vi "_backup hw-all.vi"() -> ()   [LabVIEW 2019]
uses:
  _ctrl/rw.ctl
  Capacitor/rc-seq_enum.ctl
  _ctrl/init-r-stop.ctl
  SubVIs/common/_ctrl/system-status.ctl
  _ctrl/Sinple-sequence-type.ctl
  SubVIs/common/hw-control.ctl
  common/UI.ctl
  _ctrl/create-rw-close.ctl
  _ctrl/start.ctl
  Devices/DL950/query type.ctl
  common/Global 1.vi
  81cc3607-908d-4f29-9377-88d8534cc897.vi
  716c5298-81ca-4b46-9759-33d23efd1b7f.vi
  5a08cc20-1eea-4034-90c3-b73213eb6239.vi
panel:
  out "appended array":dbl[](array[numeric])
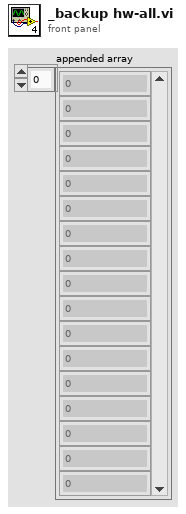
[diagram p1: front panel]
types:
  T1 = typedef "rw.ctl" = enum16{"read", "write"}
  T2 = typedef "Sinple-sequence-type.ctl" = enum16{"Register", "RC", "B1", "B2", "B3"}
  T3 = typedef "system-status.ctl" = enum16{"Initial", "Update", "Clear", "Read"}
  T4 = typedef "init-r-stop.ctl" = enum16{"ini", "read", "stop"}
  T5 = typedef "hw-control.ctl" = enum16{"DL950 ready", "DL950 clear", "DL950 trigger", "DL950 read", "DL950 read seq", "DL950 Tsingle query", "AO 12v", "AO wave", "AO 0v", "relay all-off", "Discharge check", "Discharge", "Relay1", "Relay2", "Relay3", "Relay4", "Relay5", "Relay6", "BP4610 onoff", "BP4610 set", "DSP1500 set", "DSP1500 onoff"}
  T6 = typedef "UI.ctl" = enum16{"Alarm yellow", "DL950 graph show", "DL950 graph clear", "AO value", "AO blink onoff", "Discharge relay", "Input Power", "Outpower", "Relay in1", "Relay in2", "Relay in3", "Relay in4", "Relay in5", "Relay in6", "Relay out1", "Relay out2", "Relay out3", "Relay out4", "Relay out5", "Relay out6", "Relay all off"}
  T7 = typedef "start.ctl" = enum16{"init", "open", "set", "start", "stop", "read", "read_items", "query", "close", "T_single", "reset", "exit"}
  T8 = typedef "create-rw-close.ctl" = enum16{"create", "write", "read", "close"}
  T9 = typedef "query type.ctl" = enum16{"clear", "capacitor set", "capacitor get"}
  T10 = typedef "cap_config.ctl" = cluster{"제어 전압[V]":dbl, "출력전압[V]":dbl, "전류[A]":dbl, "출력전류[A]":dbl, "ON[초]":dbl, "OFF[초]":dbl, "방전 진단[V]":dbl, "전압98[초]":dbl, "전압63[초]":dbl, "전류37[초]":dbl, "방전 시간[초]":dbl, "전압98[+/-%]":dbl, "전압63[+/-%]":dbl, "전류37[+/-%]":dbl}
  T11 = typedef "rc-seq_enum.ctl" = enum16{"hw set", "Pwr-in on", "ch-relay on", "Pwr-out on", "AO on", "AO 0v", "Pwr-in off", "Relay-all off", "Pwr-out off", "Discharge", "950 read"}
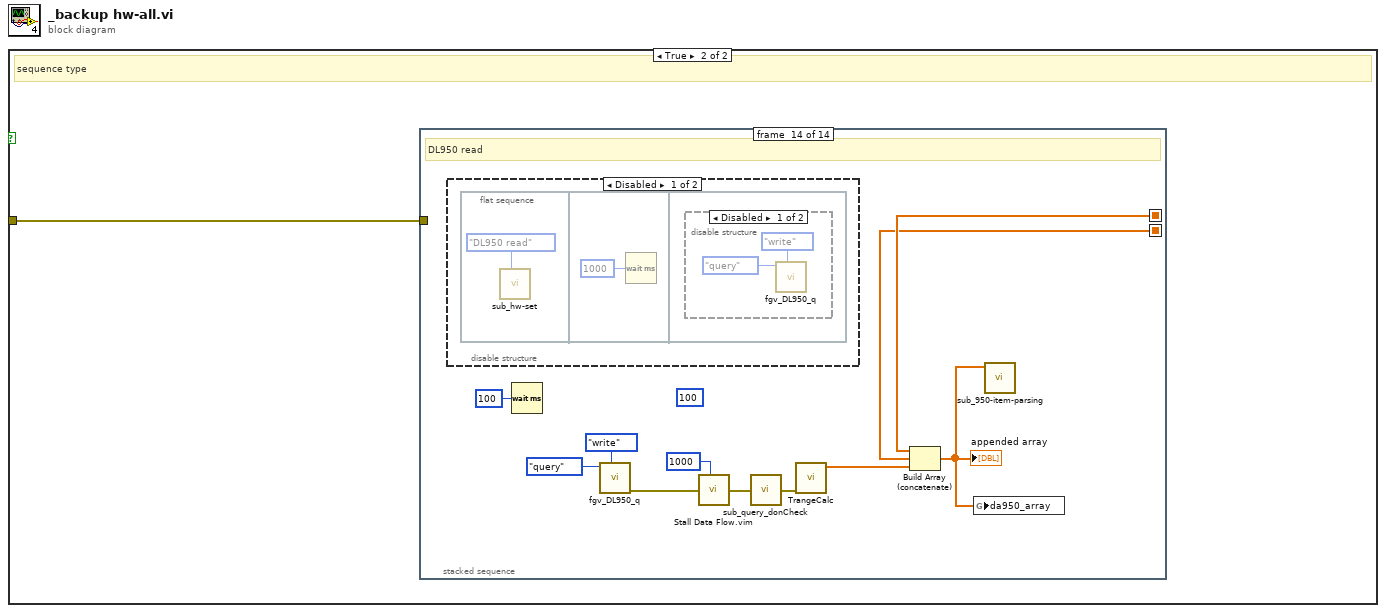
[diagram p0: block diagram]
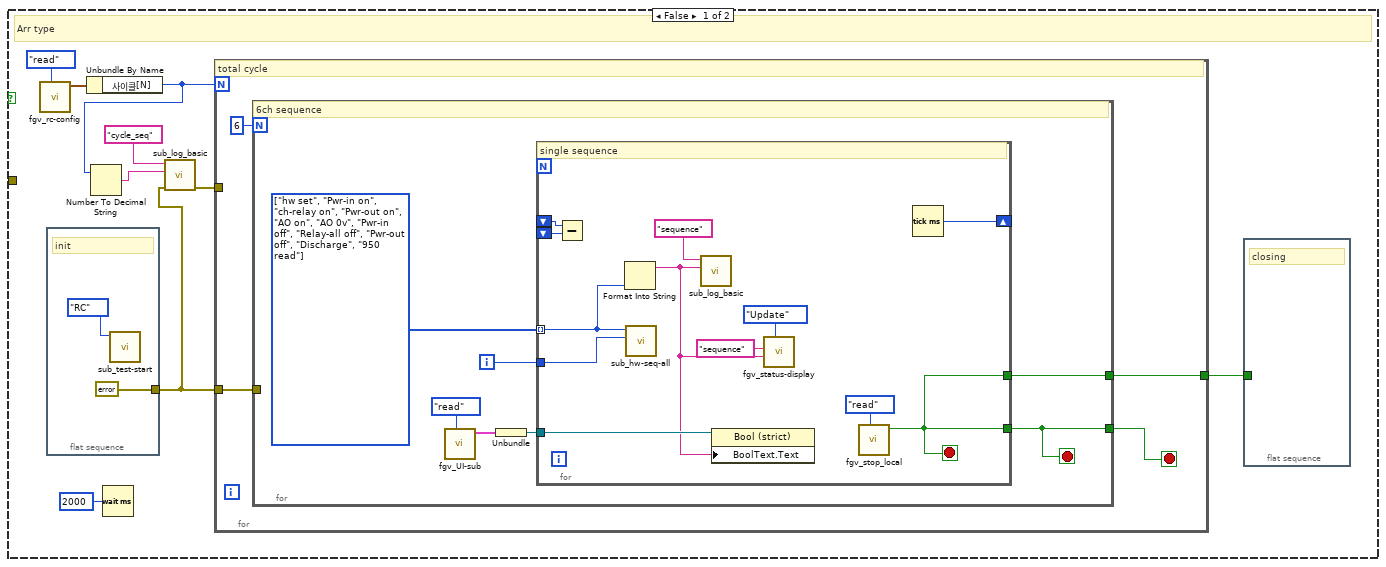
[diagram p2: hidden frame]
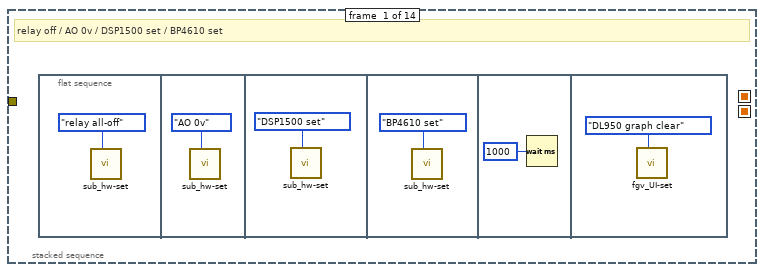
[diagram p3: hidden frame]
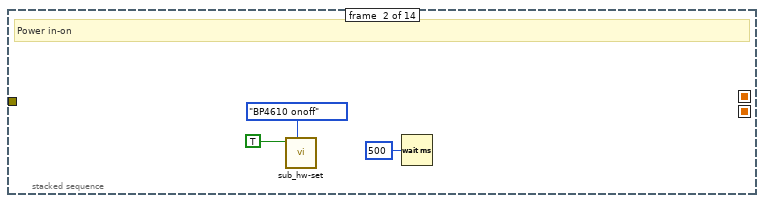
[diagram p4: hidden frame]
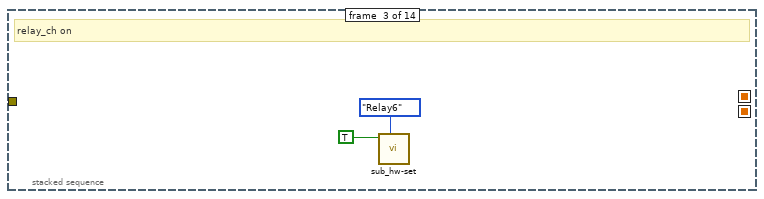
[diagram p5: hidden frame]
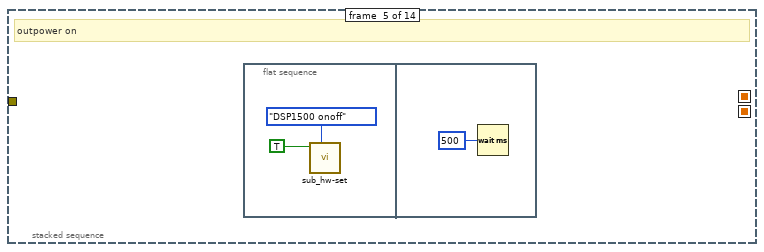
[diagram p7: hidden frame]
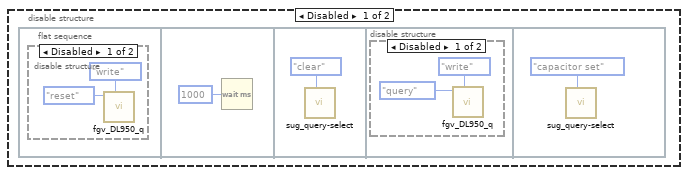
[diagram p9: hidden frame]
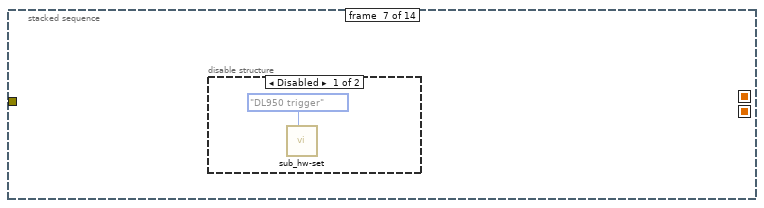
[diagram p12: hidden frame]
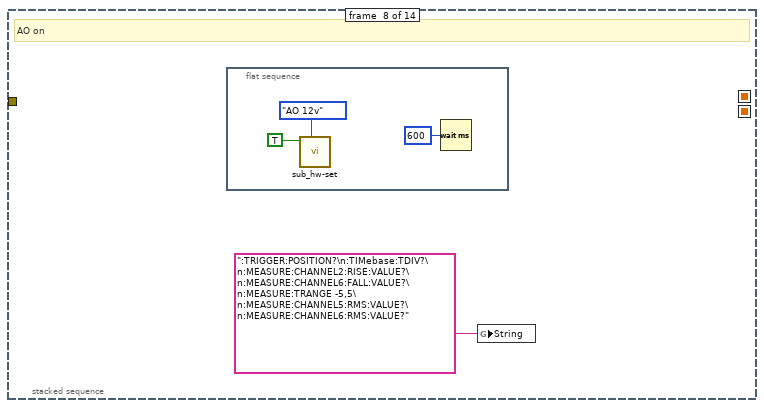
[diagram p14: hidden frame]
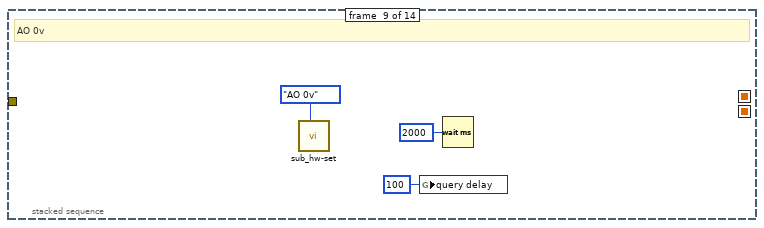
[diagram p15: hidden frame]
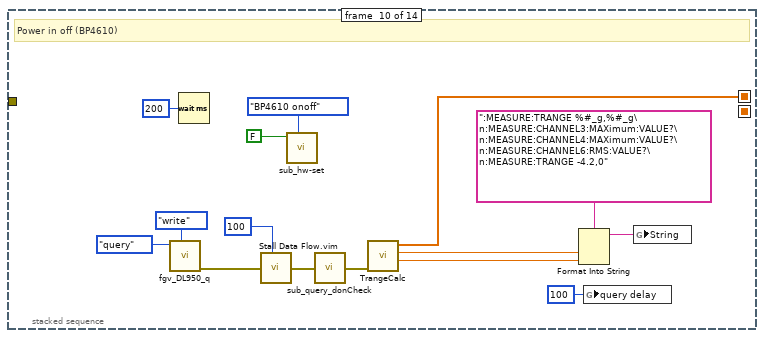
[diagram p16: hidden frame]
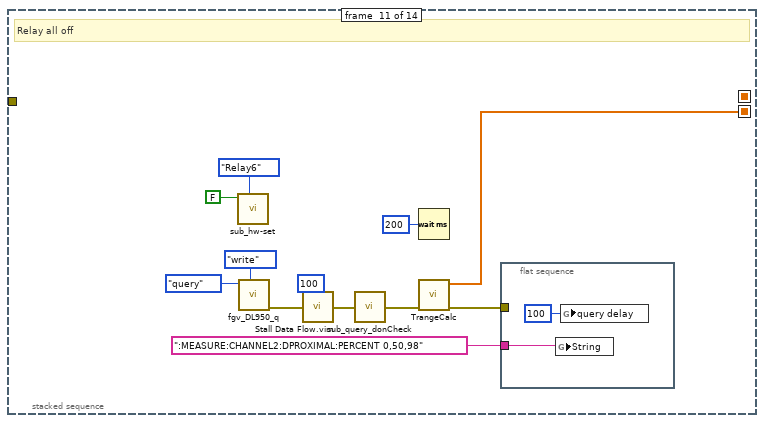
[diagram p17: hidden frame]
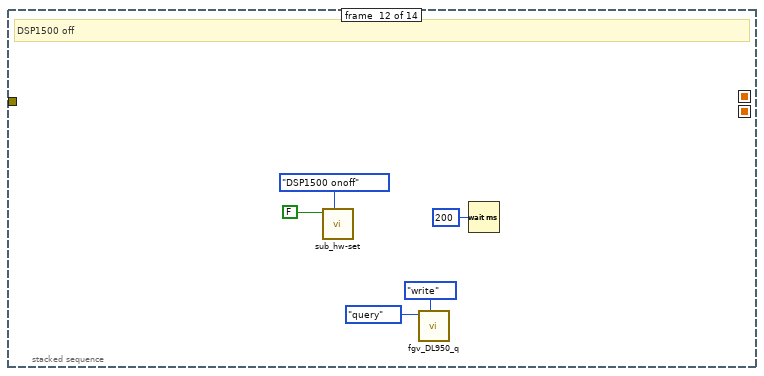
[diagram p18: hidden frame]
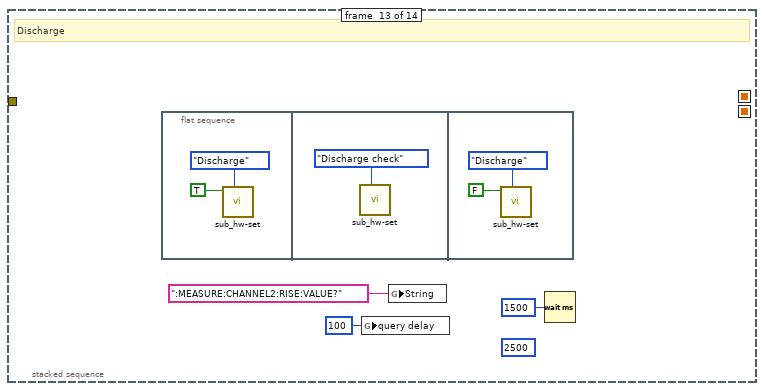
[diagram p19: hidden frame]
diagram:
  n1 = case shown="True" {
    selector: _ -> [_ _]
    tunnel: _ -> [_ w35]
    frame False {
      # "Arr type"
      n2 = call "fgv_rc-config.vi"("cmd"=rw."read") -> ("CapTestConfig 2"=w8:T10)  [unwired: 10 in]
      n3 = flat-sequence {
        tunnel: [errorcluster {"status"=FALSE, "code"=0, "source"=""} ("error constant")] -> w1
        frame #0 {
          # "init"
          n4 = call "sub_test-start.vi"(11:Sinple-sequence-type."RC" ("Type")) -> ()  [unwired: 10 in, 1 out]
        }
      }
      n5 = Unbundle By Name(w8) -> ("사이클[N]"=w4:u32)
      n6 = Number To Decimal String(number=w4) -> (decimal integer string=w3:string)  [unwired: 1 in]
      n7 = Wait (ms)(milliseconds to wait=u32 2000) -> ()  [unwired: 1 out]
      n8 = call "sub_log_basic.vi"("error in"=w1, "desc"=w3, "Title"="cycle_seq") -> ("error out"=w2:errorcluster)  [unwired: 8 in]
      n9 = for {
        N: w4 -> [_]
        tunnel: [w14] -> w7
        tunnel: w1 -> [w13]
        tunnel: w2 -> [_]
        stop <- w12 stop-if-true
        # "total cycle"
        n10 = for {
          N: 6 -> [_]
          tunnel: [w21] -> w14
          tunnel: w13 -> [_]
          tunnel: [w20] -> w12
          i -> [w16]
          stop <- w20 stop-if-true
          w22 = T11[] [enum."hw set", enum."Pwr-in on", enum."ch-relay on", enum."Pwr-out on", enum."AO on", enum."AO 0v", enum."Pwr-in off", enum."Relay-all off", enum."Pwr-out off", enum."Discharge", enum."950 read"] items=["hw set", "Pwr-in on", "ch-relay on", "Pwr-out on", "AO on", "AO 0v", "Pwr-in off", "Relay-all off", "Pwr-out off", "Discharge", "950 read"]
          # "6ch sequence"
          n11 = call "fgv_UI-sub.vi"("cmd"=rw."read") -> ("output cluster 2"=w18:cluster{"Operation stutus":refnum<vi>})  [unwired: 9 in, 1 out]
          n12 = Unbundle(w18) -> ("Operation stutus"=w17:refnum<vi>)
          n13 = for {
            tunnel: w22 -> [w29] mode=indexing
            tunnel: [w30] -> w21
            shift-right: [w34] -> _
            shift-left: _ -> [w33]
            shift-left: _ -> [w32]
            tunnel: [w30] -> w20
            tunnel: w17 -> [w25]
            tunnel: w16 -> [w23]
            stop <- w30 stop-if-true
            # "single sequence"
            n14 = Subtract(x=w33, y=w32) -> ()  [unwired: 1 out]
            n15 = Format Into String(w29) -> (resulting string=w24:string)  [unwired: 3 in, 1 out]
            n16 = call "sub_hw-seq-all.vi"("DUT Ch"=w23, "rc-sequence"=w29) -> ()  [unwired: 10 in]
            n17 = call "sub_log_basic.vi"("desc"=w24, "Title"="sequence") -> ()  [unwired: 9 in, 1 out]
            n18 = property class="Bool (strict)"(reference=w25, "BoolText.Text"=w24) -> ()  [unwired: 1 in, 2 out]
            n19 = call "fgv_status-display.vi"("Mode"=system-status."Update", "detail"=w24, "title"="sequence") -> ()  [unwired: 8 in, 1 out]
            n20 = call "fgv_stop_local.vi"("cmd"=init-r-stop."read") -> ("stop"=w30:bool)  [unwired: 10 in]
            n21 = Tick Count (ms)() -> (millisecond timer value=w34:u32)
          }
        }
      }
      n22 = flat-sequence {
        tunnel: w7 -> [_]
        frame #0 {
          # "closing"
        }
      }
    }
    frame True {
      # "sequence type"
      n23 = stacked-sequence {
        seq-local: [_ _ _ _ _ _ _ _ _ w68 _ _ _ _] -> [_ _ _ _ _ _ _ _ _ _ _ _ _ w113]
        seq-local: [_ _ _ _ _ _ _ _ _ _ w84 _ _ _] -> [_ _ _ _ _ _ _ _ _ _ _ _ _ w112]
        tunnel: w35 -> [_ _ _ _ _ _ _ _ _ _ _ _ _ _]
        frame #0 {
          # "relay off / AO 0v / DSP1500 set / BP4610 set"
          n24 = flat-sequence {
            frame #0 {
              n25 = call "sub_hw-set.vi"("cmd"=hw-control."relay all-off") -> ()  [unwired: 10 in, 1 out]
            }
            frame #1 {
              n26 = call "sub_hw-set.vi"("cmd"=hw-control."AO 0v") -> ()  [unwired: 10 in, 1 out]
            }
            frame #2 {
              n27 = call "sub_hw-set.vi"("cmd"=hw-control."DSP1500 set") -> ()  [unwired: 10 in, 1 out]
            }
            frame #3 {
              n28 = call "sub_hw-set.vi"("cmd"=hw-control."BP4610 set") -> ()  [unwired: 10 in, 1 out]
            }
            frame #4 {
              n29 = Wait (ms)(milliseconds to wait=u32 1000) -> ()  [unwired: 1 out]
            }
            frame #5 {
              n30 = call "fgv_UI-set.vi"("cmd"=UI."DL950 graph clear") -> ()  [unwired: 10 in, 1 out]
            }
          }
        }
        frame #1 {
          # "Power in-on"
          n31 = call "sub_hw-set.vi"("cmd"=hw-control."BP4610 onoff", "onoff"=TRUE) -> ()  [unwired: 9 in, 1 out]
          n32 = Wait (ms)(milliseconds to wait=u32 500) -> ()  [unwired: 1 out]
        }
        frame #2 {
          # "relay_ch on"
          n33 = call "sub_hw-set.vi"("cmd"=hw-control."Relay6", "onoff"=TRUE) -> ()  [unwired: 9 in, 1 out]
        }
        frame #3 {
          # "-"
        }
        frame #4 {
          # "outpower on"
          n34 = flat-sequence {
            frame #0 {
              n35 = call "sub_hw-set.vi"("cmd"=hw-control."DSP1500 onoff", "onoff"=TRUE) -> ()  [unwired: 9 in, 1 out]
            }
            frame #1 {
              n36 = Wait (ms)(milliseconds to wait=u32 500) -> ()  [unwired: 1 out]
            }
          }
        }
        frame #5 {
          # "DL950 clear item"
          n37 = disable-structure shown="Enabled" {
            frame Disabled {
              n38 = flat-sequence {
                frame #0 {
                  n39 = disable-structure shown="Disabled" {
                    frame Disabled {
                      n40 = call "fgv_DL950_q.vi"("cmd"=create-rw-close."write", "data"=start."reset") -> ()  [unwired: 8 in, 2 out]
                    }
                    frame Enabled {
                    }
                  }
                }
                frame #1 {
                  n41 = Wait (ms)(milliseconds to wait=u32 1000) -> ()  [unwired: 1 out]
                }
                frame #2 {
                  n42 = call "sug_query-select.vi"("query type"=query_type."clear") -> ()  [unwired: 11 in]
                }
                frame #3 {
                  n43 = disable-structure shown="Disabled" {
                    frame Disabled {
                      n44 = call "fgv_DL950_q.vi"("cmd"=create-rw-close."write", "data"=start."query") -> ()  [unwired: 8 in, 2 out]
                    }
                    frame Enabled {
                    }
                  }
                }
                frame #4 {
                  n45 = call "sug_query-select.vi"("query type"=query_type."capacitor set") -> ()  [unwired: 11 in]
                }
              }
            }
            frame Enabled {
            }
          }
        }
        frame #6 {
          n46 = disable-structure shown="Disabled" {
            frame Disabled {
              n47 = call "sub_hw-set.vi"("cmd"=hw-control."DL950 trigger") -> ()  [unwired: 10 in, 1 out]
            }
            frame Enabled {
            }
          }
        }
        frame #7 {
          # "AO on"
          n48 = flat-sequence {
            frame #0 {
              n49 = call "sub_hw-set.vi"("cmd"=hw-control."AO 12v", "onoff"=TRUE) -> ()  [unwired: 9 in, 1 out]
              n50 = Wait (ms)(milliseconds to wait=u32 600) -> ()  [unwired: 1 out]
            }
          }
          n51 = global write "Global 1.vi" "String"(":TRIGGER:POSITION?\n:TIMebase:TDIV?\n:MEASURE:CHANNEL2:RISE:VALUE?\n:MEASURE:CHANNEL6:FALL:VALUE?\n:MEASURE:TRANGE -5,5\n:MEASURE:CHANNEL5:RMS:VALUE?\n:MEASURE:CHANNEL6:RMS:VALUE?" ("String")) -> ()
        }
        frame #8 {
          # "AO 0v"
          n52 = call "sub_hw-set.vi"("cmd"=hw-control."AO 0v") -> ()  [unwired: 10 in, 1 out]
          n53 = global write "Global 1.vi" "query delay"(u32 100 ("query delay")) -> ()
          n54 = Wait (ms)(milliseconds to wait=u32 2000) -> ()  [unwired: 1 out]
        }
        frame #9 {
          # "Power in off (BP4610)"
          n55 = call "fgv_DL950_q.vi"("cmd"=create-rw-close."write", "data"=start."query") -> ("error out"=w67:errorcluster)  [unwired: 8 in, 1 out]
          n56 = Wait (ms)(milliseconds to wait=u32 200) -> ()  [unwired: 1 out]
          n57 = call "Stall Data Flow.vim"("value in"=w67, "dt"=u32 100 ("milliseconds to wait")) -> ("value out"=w65:errorcluster)  [unwired: 1 out]
          n58 = call "sub_hw-set.vi"("cmd"=hw-control."BP4610 onoff", "onoff"=FALSE) -> ()  [unwired: 9 in, 1 out]
          n59 = call "sub_query_donCheck.vi"("error in (no error)"=w65) -> ("error out"=w69:errorcluster)  [unwired: 2 in]
          n60 = call "TrangeCalc.vi"("error in (no error)"=w69) -> ("T2"=w73:dbl, "T1"=w72:dbl, "array"=w68:dbl[])  [unwired: 6 in, 1 out]
          n61 = Format Into String(format string=":MEASURE:TRANGE %#_g,%#_g\n:MEASURE:CHANNEL3:MAXimum:VALUE?\n:MEASURE:CHANNEL4:MAXimum:VALUE?\n:MEASURE:CHANNEL6:RMS:VALUE?\n:MEASURE:TRANGE -4.2,0", w72, w73) -> (resulting string=w74:string)  [unwired: 2 in, 1 out]
          n62 = global write "Global 1.vi" "query delay"(u32 100 ("query delay")) -> ()
          n63 = global write "Global 1.vi" "String"(w74) -> ()
        }
        frame #10 {
          # "Relay all off"
          n64 = call "sub_hw-set.vi"("cmd"=hw-control."Relay6", "onoff"=FALSE) -> ()  [unwired: 9 in, 1 out]
          n65 = call "fgv_DL950_q.vi"("cmd"=create-rw-close."write", "data"=start."query") -> ("error out"=w86:errorcluster)  [unwired: 8 in, 1 out]
          n66 = call "Stall Data Flow.vim"("value in"=w86, "dt"=u32 100 ("milliseconds to wait")) -> ("value out"=w80:errorcluster)  [unwired: 1 out]
          n67 = call "sub_query_donCheck.vi"("error in (no error)"=w80) -> ("error out"=w85:errorcluster)  [unwired: 2 in]
          n68 = Wait (ms)(milliseconds to wait=u32 200) -> ()  [unwired: 1 out]
          n69 = call "TrangeCalc.vi"("error in (no error)"=w85) -> ("error out"=w83:errorcluster, "array"=w84:dbl[])  [unwired: 6 in, 2 out]
          n70 = flat-sequence {
            tunnel: w83 -> [_]
            tunnel: ":MEASURE:CHANNEL2:DPROXIMAL:PERCENT 0,50,98" ("format string") -> [w93]
            frame #0 {
              n71 = global write "Global 1.vi" "String"(w93) -> ()
              n72 = global write "Global 1.vi" "query delay"(u32 100 ("query delay")) -> ()
            }
          }
        }
        frame #11 {
          # "DSP1500 off"
          n73 = call "sub_hw-set.vi"("cmd"=hw-control."DSP1500 onoff", "onoff"=FALSE) -> ()  [unwired: 9 in, 1 out]
          n74 = call "fgv_DL950_q.vi"("cmd"=create-rw-close."write", "data"=start."query") -> ()  [unwired: 8 in, 2 out]
          n75 = Wait (ms)(milliseconds to wait=u32 200) -> ()  [unwired: 1 out]
        }
        frame #12 {
          (unwired) u32 2500 ("milliseconds to wait")
          # "Discharge"
          n76 = flat-sequence {
            frame #0 {
              n77 = call "sub_hw-set.vi"("cmd"=hw-control."Discharge", "onoff"=TRUE) -> ()  [unwired: 9 in, 1 out]
            }
            frame #1 {
              n78 = call "sub_hw-set.vi"("cmd"=hw-control."Discharge check") -> ()  [unwired: 10 in, 1 out]
            }
            frame #2 {
              n79 = call "sub_hw-set.vi"("cmd"=hw-control."Discharge", "onoff"=FALSE) -> ()  [unwired: 9 in, 1 out]
            }
          }
          n80 = global write "Global 1.vi" "query delay"(u32 100 ("query delay")) -> ()
          n81 = global write "Global 1.vi" "String"(":MEASURE:CHANNEL2:RISE:VALUE?" ("format string")) -> ()
          n82 = Wait (ms)(milliseconds to wait=u32 1500) -> ()  [unwired: 1 out]
        }
        frame #13 {
          (unwired) u32 100 ("milliseconds to wait")
          # "DL950 read"
          n83 = disable-structure shown="Disabled" {
            frame Disabled {
              n84 = flat-sequence {
                frame #0 {
                  n85 = call "sub_hw-set.vi"("cmd"=hw-control."DL950 read") -> ()  [unwired: 10 in, 1 out]
                }
                frame #1 {
                  n86 = Wait (ms)(milliseconds to wait=u32 1000) -> ()  [unwired: 1 out]
                }
                frame #2 {
                  n87 = disable-structure shown="Disabled" {
                    frame Disabled {
                      n88 = call "fgv_DL950_q.vi"("cmd"=create-rw-close."write", "data"=start."query") -> ()  [unwired: 8 in, 2 out]
                    }
                    frame Enabled {
                    }
                  }
                }
              }
            }
            frame Enabled {
            }
          }
          n89 = Wait (ms)(milliseconds to wait=u32 100) -> ()  [unwired: 1 out]
          n90 = call "fgv_DL950_q.vi"("cmd"=create-rw-close."write", "data"=start."query") -> ("error out"=w114:errorcluster)  [unwired: 8 in, 1 out]
          n91 = call "Stall Data Flow.vim"("value in"=w114, "dt"=u32 1000 ("milliseconds to wait")) -> ("value out"=w109:errorcluster)  [unwired: 1 out]
          n92 = call "sub_query_donCheck.vi"("error in (no error)"=w109) -> ("error out"=w108:errorcluster)  [unwired: 2 in]
          n93 = call "TrangeCalc.vi"("error in (no error)"=w108) -> ("array"=w111:dbl[])  [unwired: 6 in, 3 out]
          n94 = Build Array (concatenate)(w113, w112, w111) -> (w107:dbl[])
          "appended array" <- w107
          n95 = global write "Global 1.vi" "da950_array"(w107) -> ()
          n96 = call "sub_950-item-parsing.vi"("950 result arr"=w107) -> ()  [unwired: 11 in]
        }
      }
    }
  }
